vi "LVProjectShortcut_StoreFileSelectionMode.vi"(7 "VI Refnum":refnum<vi>, 8 "error in":errorcluster, 10 "files in libraries":bool, 11 "Ctl Refnum":refnum<vi>) -> (0 "error out":errorcluster, 2 "Selection Mode":T1(ring))   [LabVIEW 2017, in "LVProject Shortcut.lvlib"]
doc: "Stores the <b>files in libraries</b> as Object Tag of the <b>Ctl Refnum</b>. This VI saves the VI specified by the <b>VI Refnum</b>.\n\nIf <b>VI Refnum</b> is invalide, this VI saves the caller VI."
uses:
  LVProject Shortcut.lvlib
  <vilib>/UserTags/UserTags.lvlib
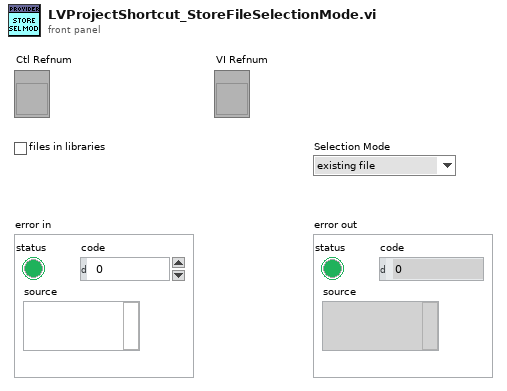
[diagram p1: front panel]
types:
  T1 = enum32{"existing file", "new file", "new or existing file", "existing dir", "new dir", "new or existing dir", "existing file (use LLBs)", "new file (use LLBs)", "new or existing file (use LLBs)", "new or existing file or directory (use LLBs)", "existing dir (use LLBs)", "new dir (use LLBs)", "new or existing dir (use LLBs)", "existing file or dir", "new file or dir", "new or existing file or dir", "existing file or dir (use LLBs)", "new file or dir (use LLBs)"}
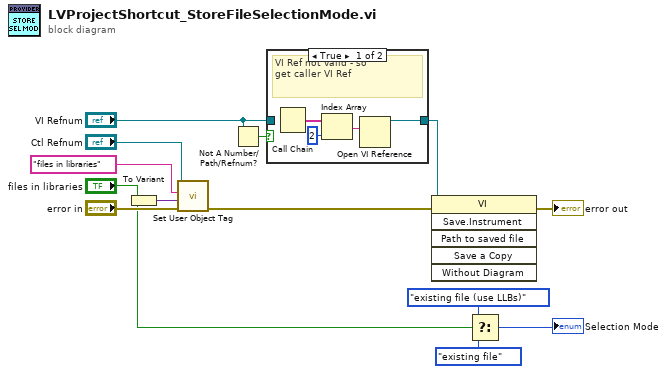
[diagram p0: block diagram]
diagram:
  n1 = To Variant(anything="files in libraries") -> (Variant=w10:variant)
  n2 = call <vilib>:"Set User Object Tag.vi"("error in (no error)"="error in", "Value"=w10, "Tag Name"="files in libraries", "Generic Refnum"="Ctl Refnum") -> ("error out"=w9:errorcluster)  [unwired: 5 in, 2 out]
  n3 = Not A Number/Path/Refnum?(number/path/refnum="VI Refnum") -> (NaN/Path/Refnum?=w7:bool)
  n4 = case shown="True" w7 {
    tunnel: [w14 w18] -> w6
    tunnel: "VI Refnum" -> [_ w18]
    frame True {
      # "VI Ref not valid - so\nget caller VI Ref"
      n5 = Call Chain() -> (call chain=w16:string[])
      n6 = Index Array(array=w16, index=2 ("Index")) -> (element=w17:string)
      n7 = Open VI Reference(vi path=w17) -> (vi reference=w14:refnum<vi>)  [unwired: 5 in, 1 out]
    }
    frame False {
      # "VI Ref valid - so\npass it"
    }
  }
  n8 = invoke class="VI" method="Save.Instrument"(reference=w6, error in=w9) -> (error out=→"error out":errorcluster)  [unwired: 4 in, 5 out]
  n9 = Select(t=T1."existing file (use LLBs)" ("Browse Options:Selection Mode"), s="files in libraries", f=T1."existing file" ("Browse Options:Selection Mode")) -> (s? t:f=→"Selection Mode":T1)
